vi "json_get_names.vi"(8 "error in (no error)":errorcluster, 11 "variant in":variant) -> (0 "error out":errorcluster, 1 "values":variant[](array[variant]), 2 "names":string[](array[string]), 3 "variant out":variant)   [LabVIEW 2017, in "rethinkdb.lvlib"]
uses:
  rethinkdb.lvlib
  <vilib>/Utility/Data Type/NI_Data Type.lvlib
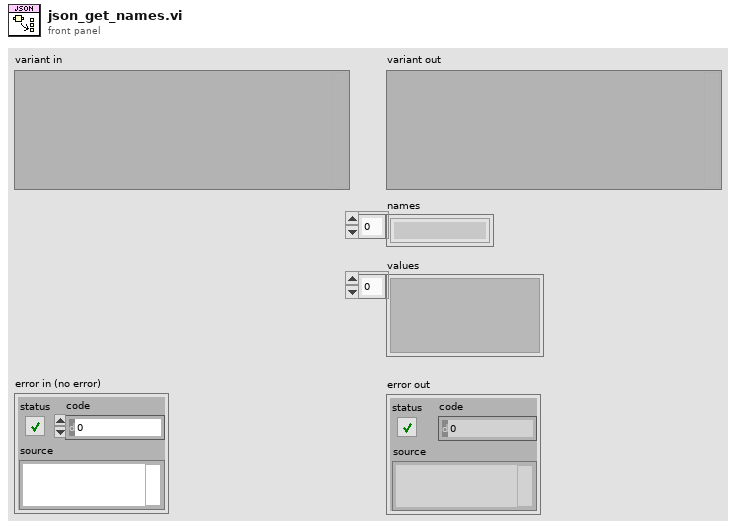
[diagram p1: front panel]
types:
  T1 = typedef "NI_Data Type.lvlib/Data Type.ctl" = enum8{"Invalid Type", "Void", "I8", "I16", "I32", "I64", "U8", "U16", "U32", "U64", "Single Float", "Double Float", "Extended Float", "Single Complex", "Double Complex", "Extended Complex", "Enum U8", "Enum U16", "Enum U32", "Enum U64", "Single Float With Unit", "Double Float With Unit", "Extended Float With Unit", "Single Complex with Unit", "Double Complex with Unit", "Extended Complex with Unit", "Boolean", "String", "Path", "Picture", "Tag", "Array", "Cluster", "Variant", "LV Variant", "Waveform", "Timestamp", "Digital Waveform", "Digital Data", "ExpressData", "Refnum", "External Data", "VI", "Poly VI", "LabVIEW Class Instance", "Fixed Point"}
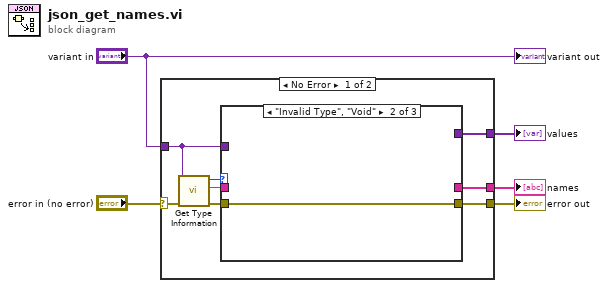
[diagram p0: block diagram]
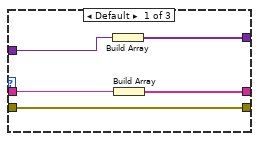
[diagram p2: hidden frame]
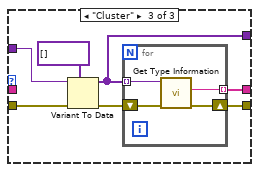
[diagram p3: hidden frame]
diagram:
  n1 = case shown="No Error" "error in (no error)" {
    selector: "error in (no error)" -> [w13 w31]
    tunnel: [w11 w31] -> w4
    tunnel: "variant in" -> [w10 _]
    tunnel: [w7 _] -> w2
    tunnel: [w6 _] -> w1
    frame No Error {
      n2 = call <vilib>:"Get Type Information.vi"("error in (no error)"=w13, "Variant"=w10) -> ("error out"=w12:errorcluster, "Name"=w8:string, "Type"=w9:T1)  [unwired: 5 in, 2 out]
      n3 = case shown="\"Invalid Type\", \"Void\"" w9 {
        tunnel: w12 -> [w16 w19 w26]
        tunnel: [w16 w19 w22] -> w11
        tunnel: w10 -> [w15 _ w24]
        tunnel: w8 -> [w18 _ _]
        tunnel: [w17 _ w21] -> w6
        tunnel: [w14 _ w20] -> w7
        frame Default {
          n4 = Build Array(w15) -> (w14:variant[])
          n5 = Build Array(w18) -> (w17:string[])
        }
        frame "Invalid Type", "Void" {
        }
        frame "Cluster" {
          n6 = Variant To Data(error in=w26, type=variant[] [], Variant=w24) -> (data=w20:variant[], error out=w23:errorcluster)
          n7 = for {
            tunnel: w20 -> [w29] mode=indexing
            shift-right: [w28] -> w22
            shift-left: w23 -> [w30]
            tunnel: [w27] -> w21 mode=indexing
            n8 = call <vilib>:"Get Type Information.vi"("error in (no error)"=w30, "Variant"=w29) -> ("error out"=w28:errorcluster, "Name"=w27:string)  [unwired: 5 in, 3 out]
          }
        }
      }
    }
    frame Error {
    }
  }
  "error out" <- w4
  "names" <- w1
  "values" <- w2
  "variant out" <- "variant in"
